vi "testEvtDetailsToJSON.vi"(8 "error in (no error)":errorcluster) -> (0 "error out":errorcluster)   [LabVIEW 2018]
doc: "Test the evtDetailsToJSON.vi."
uses:
  src/TcpServer/TcpServer.lvclass
  <vilib>/addons/_JKI Toolkits/Caraya/classes/Assert/Assert Equal Value_Variant.vi
  <vilib>/addons/_JKI Toolkits/Caraya/classes/Assert/Assert Equal Value and Type_Variant.vi
  <vilib>/addons/_JKI Toolkits/Caraya/classes/Test/Test.lvclass
  <vilib>/addons/_JKI Toolkits/Caraya/classes/Assert/Assert.lvclass
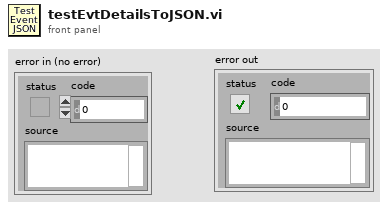
[diagram p1: front panel]
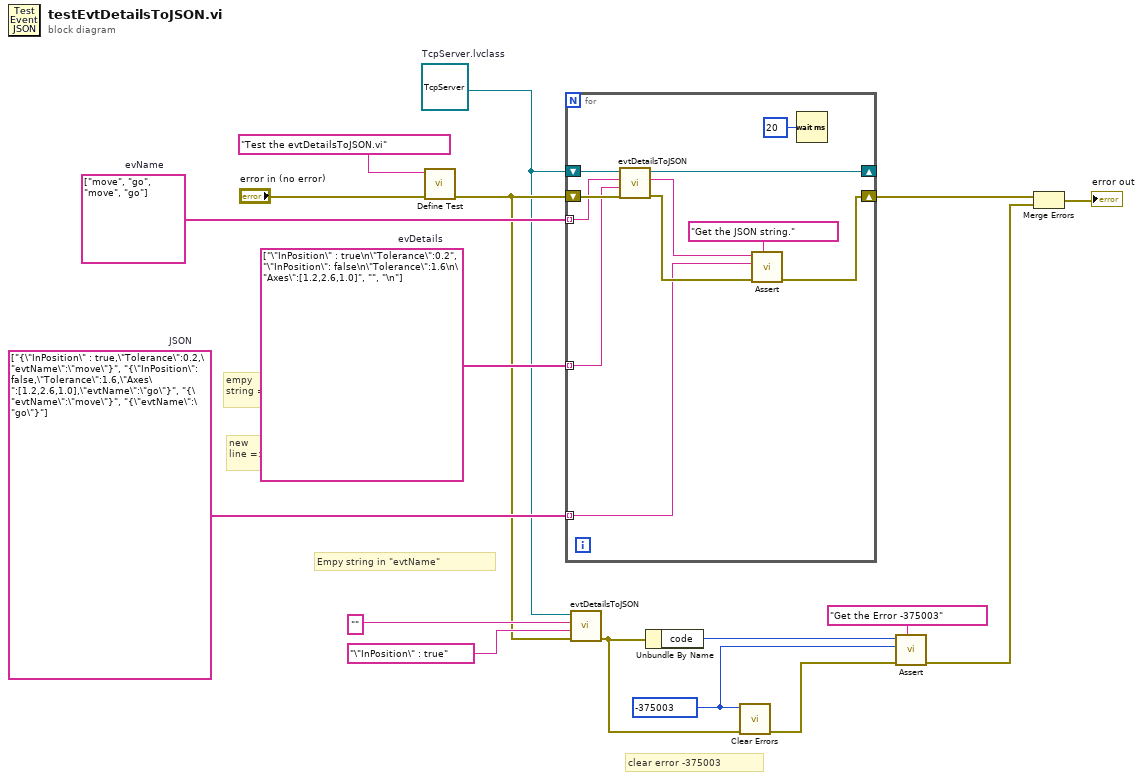
[diagram p0: block diagram]
diagram:
  w6 = -375003 ("code")
  w13 = string[] ["{\"InPosition\" : true,\"Tolerance\":0.2,\"evtName\":\"move\"}", "{\"InPosition\": false,\"Tolerance\":1.6,\"Axes\":[1.2,2.6,1.0],\"evtName\":\"go\"}", "{\"evtName\":\"move\"}", "{\"evtName\":\"go\"}"]  # JSON
  w14 = string[] ["\"InPosition\" : true\n\"Tolerance\":0.2", "\"InPosition\": false\n\"Tolerance\":1.6\n\"Axes\":[1.2,2.6,1.0]", "", "\n"]  # evDetails
  w15 = string[] ["move", "go", "move", "go"]  # evName
  w1 = refnum<class "TcpServer.lvclass"> refnum  # TcpServer.lvclass
  # "new \nline =>"
  # "empy \nstring =>"
  # "clear error -375003"
  # "Empy string in \"evtName\""
  n1 = call <vilib>:"Define Test.vi"("error in (no error)"="error in (no error)", "Label (VI Title)"="Test the evtDetailsToJSON.vi") -> ("error out"=w5:errorcluster)  [unwired: 9 in]
  n2 = for {
    tunnel: w15 -> [w26] mode=indexing
    tunnel: w14 -> [w25] mode=indexing
    tunnel: w13 -> [w18] mode=indexing
    shift-right: [w19] -> w4
    shift-left: w5 -> [w27]
    shift-right: [w21] -> _
    shift-left: w1 -> [w28]
    n3 = call "evtDetailsToJSON.vi"("error in (no error)"=w27, "evtDetails"=w25, "evtName"=w26, "TcpServer.lvclass"=w28) -> ("error out"=w20:errorcluster, "JSON string"=w22:string, "TcpServer.lvclass"=w21:refnum<class "TcpServer.lvclass">)  [unwired: 5 in]
    n4 = call-poly <vilib>:"Assert.vi"("Label"="Get the JSON string.", "error in (no error)"=w20, "Y"=w18, "X"=w22) -> ("error out"=w19:errorcluster)  [unwired: 7 in]
    n5 = Wait (ms)(milliseconds to wait=u32 20) -> ()  [unwired: 1 out]
  }
  n6 = call "evtDetailsToJSON.vi"("error in (no error)"=w5, "evtDetails"="\"InPosition\" : true" ("String"), "evtName"="" ("String"), "TcpServer.lvclass"=w1) -> ("error out"=w8:errorcluster)  [unwired: 5 in, 2 out]
  n7 = Unbundle By Name(w8) -> ("code"=w7:i32)
  n8 = call <vilib>:"Clear Errors.vi"("error in (no error)"=w8, "specific error code to clear (0: all)"=w6) -> ("error out"=w9:errorcluster)  [unwired: 4 in, 1 out]
  n9 = call-poly <vilib>:"Assert.vi"("Label"="Get the Error -375003", "error in (no error)"=w9, "Y"=w6, "X"=w7) -> ("error out"=w3:errorcluster)  [unwired: 7 in]
  n10 = Merge Errors(w4, w3) -> (→"error out":errorcluster)
